vi "Test_read_memory.vi"() -> ()   [LabVIEW 2013]
uses:
  Input_5782/5782_Fast_PID_states.ctl
  <vilib>/Platform/TimedLoop/XDataNode/timing_clust.ctl
  <vilib>/Platform/TimedLoop/XDataNode/nitl_modes.ctl
  <vilib>/Platform/TimedLoop/XDataNode/wakeup.ctl
  <vilib>/rvi/FXPMathLib/FxpConvert/subVIs/nifxpmath_Convert_SimConfig.ctl
  <vilib>/fxp/LVFixedPointQuantizationPolicyTypeDef.ctl
  <vilib>/fxp/LVFixedPointOverflowPolicyTypeDef.ctl
  <vilib>/rvi/Emulation/niFpgaSctlEmulationGetInTimedLoop.vi
  <vilib>/rvi/Emulation/niFpgaEmulationReportErrorSimple.vi
  <vilib>/rvi/Emulation/niFpgaGetClockAttributes.vi
  <vilib>/rvi/eio/common/nirviEmuTemplateMethod_errors.vi
  <vilib>/rvi/Emulation/niFpgaCriticalErrorInLSC.vi
  <vilib>/rvi/FXPMathLib/FxpConvert/simVIs/DllFxpConvertTemp_sub.vi
  <vilib>/rvi/Memory/Memory_Emulation/nirvimemoryFastEmulationFpgaImpl.vi
  <instcachedir>/0/nirvimemoryFastEmulationFpgaImpl_5FBAB50466BC4C939F684F8805638BFC.lvgen/nirvimemoryFastEmulationFpgaImpl_5FBAB50466BC4C939F684F8805638BFC_003.vi
  <vilib>/rvi/DataTransferAndStorage/Container/Common/niFpgaContainerGetUniqueNameForEmu.vi
  <vilib>/rvi/Memory/Memory_Emulation/nirvimemoryFastEmulation.vi
  <vilib>/rvi/Memory/Memory_Emulation/nirvimemoryEmulation.vi
  <vilib>/rvi/interface/RandomDataEmulation/nirviRandomDataFPGAFIFO.vi
  <vilib>/rvi/interface/RandomDataEmulation/niFpgaRandomDataHandleErrors.vi
  <vilib>/Platform/TimedLoop/XDataNode/XDataNode.xnode
  <vilib>/eio/EIONode/EIONode.xnode
  <vilib>/rvi/FXPMathLib/FxpInterpret/XNode/nifxpmath_Interpret.xnode
  <vilib>/rvi/FXPMathLib/FxpConvert/XNode/nifxpmath_Convert.xnode
  <vilib>/rvi/DataTransferAndStorage/Container/XNode/niFpgaContainer.xnode
  <vilib>/rvi/interface/RandomDataEmulation/nirviRandomDataFpgaReadWriteTemplate.vi
  <vilib>/Platform/TimedLoop/XDataNode/XDNodeRunTimeDep.lvlib
panel:
  out "IO Module\\Trigger Input":bool
  in  "Trigger Acquisition":bool
  in  "IO Module\\AO Data Sync":bool=TRUE
  in  "IO Module\\SPI Write Data":u16
  out "IO Module\\SPI Read Data":u8
  in  "IO Module\\SPI Read":bool
  in  "IO Module\\SPI Write":bool
  in  "IO Module\\SPI Address":u16
  in  "IO Module\\SPI Device":u8
  out "IO Module\\SPI Idle":bool
  in  "User Command Commit":bool
  in  "User Command":u8
  out "User Command Idle":bool
  out "User Command Status":u8
  in  "User Data 0":u8
  in  "User Data 1":u8
  out "PLL Locked":bool
  out "User Error":bool
  out "Configured?":bool
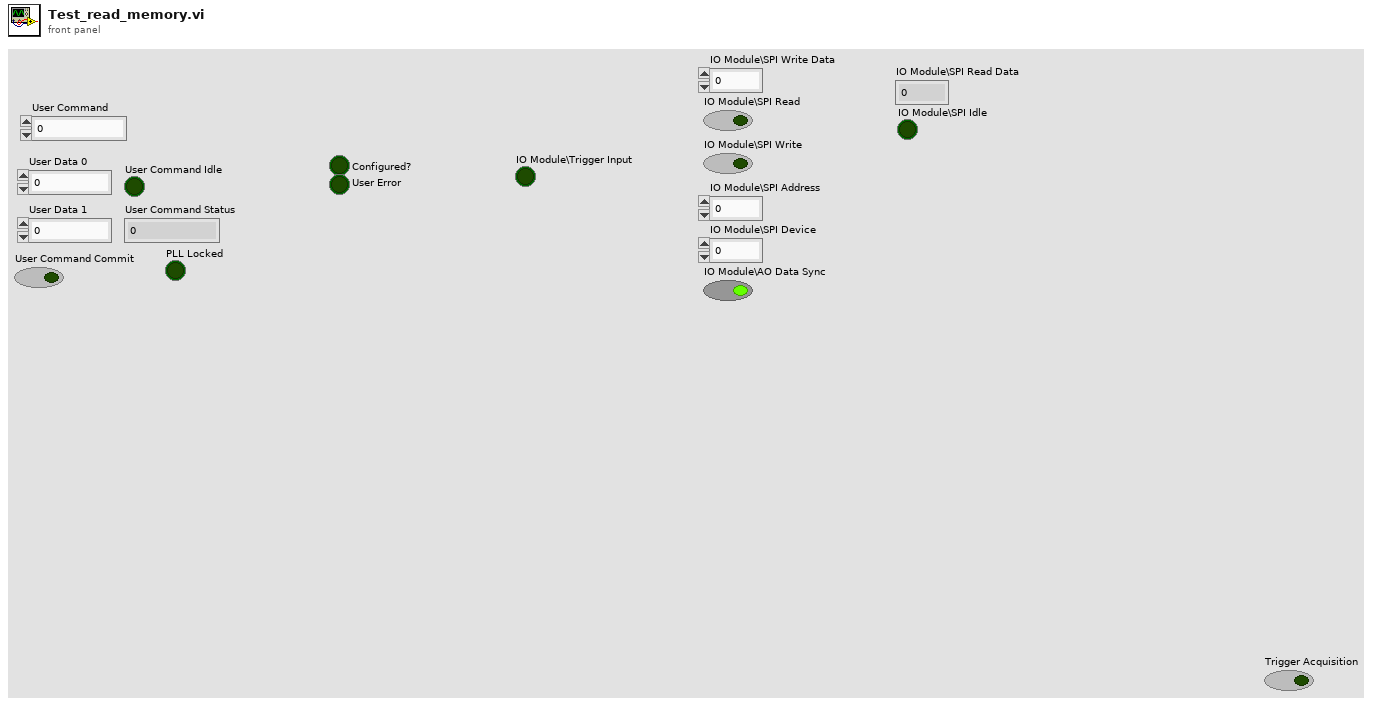
[diagram p1: front panel]
types:
  T1 = typedef "5782_Fast_PID_states.ctl" = enum8{"Wait for trigger", "Acquisition", "Send record length", "Wait for output", "Quiet period"}
  T2 = typedef "XDNodeRunTimeDep.lvlib/timing_clust.ctl" = cluster{"Expected End [f-1]":u64, "Actual End [f-1]":u64, "Finished Late? [f-1]":bool, "Expected End [i-1]":u64, "Actual End [i-1]":u64, "Finished Late? [i-1]":bool, "Expected Start [i]":u64, "Actual Start [i]":u64, "Expected Start [f]":u64, "Actual Start [f]":u64, "Source Name":string, "Structure Name":string, "Period":i64, "Deadline":i64, "Offset":i64, "Start":i64, "Priority":i32, "Timeout":i32, "Mode":T3, "Wakeup Reason":T4, "Error":errorcluster, "Source Type":string, "Secondary Source Type":string, "Global End Time":u64, "Global Start Time":u64, "Frame Duration":u64, "Iteration Duration":u64, "Assigned CPU":i32, "I/O Scan Engine Mode":u32}
  T3 = typedef "XDNodeRunTimeDep.lvlib/nitl_modes.ctl" = enum32{"No Change", "Process missed periods, maintain original phase", "Discard missed periods, maintain original phase", "Process missed periods, ignore original phase", "Discard missed periods, ignore original phase"}
  T4 = typedef "XDNodeRunTimeDep.lvlib/wakeup.ctl" = enum32{"Normal", "Aborted", "Asynchronous wakeup", "Timing source error", "Timed loop error", "Timeout"}
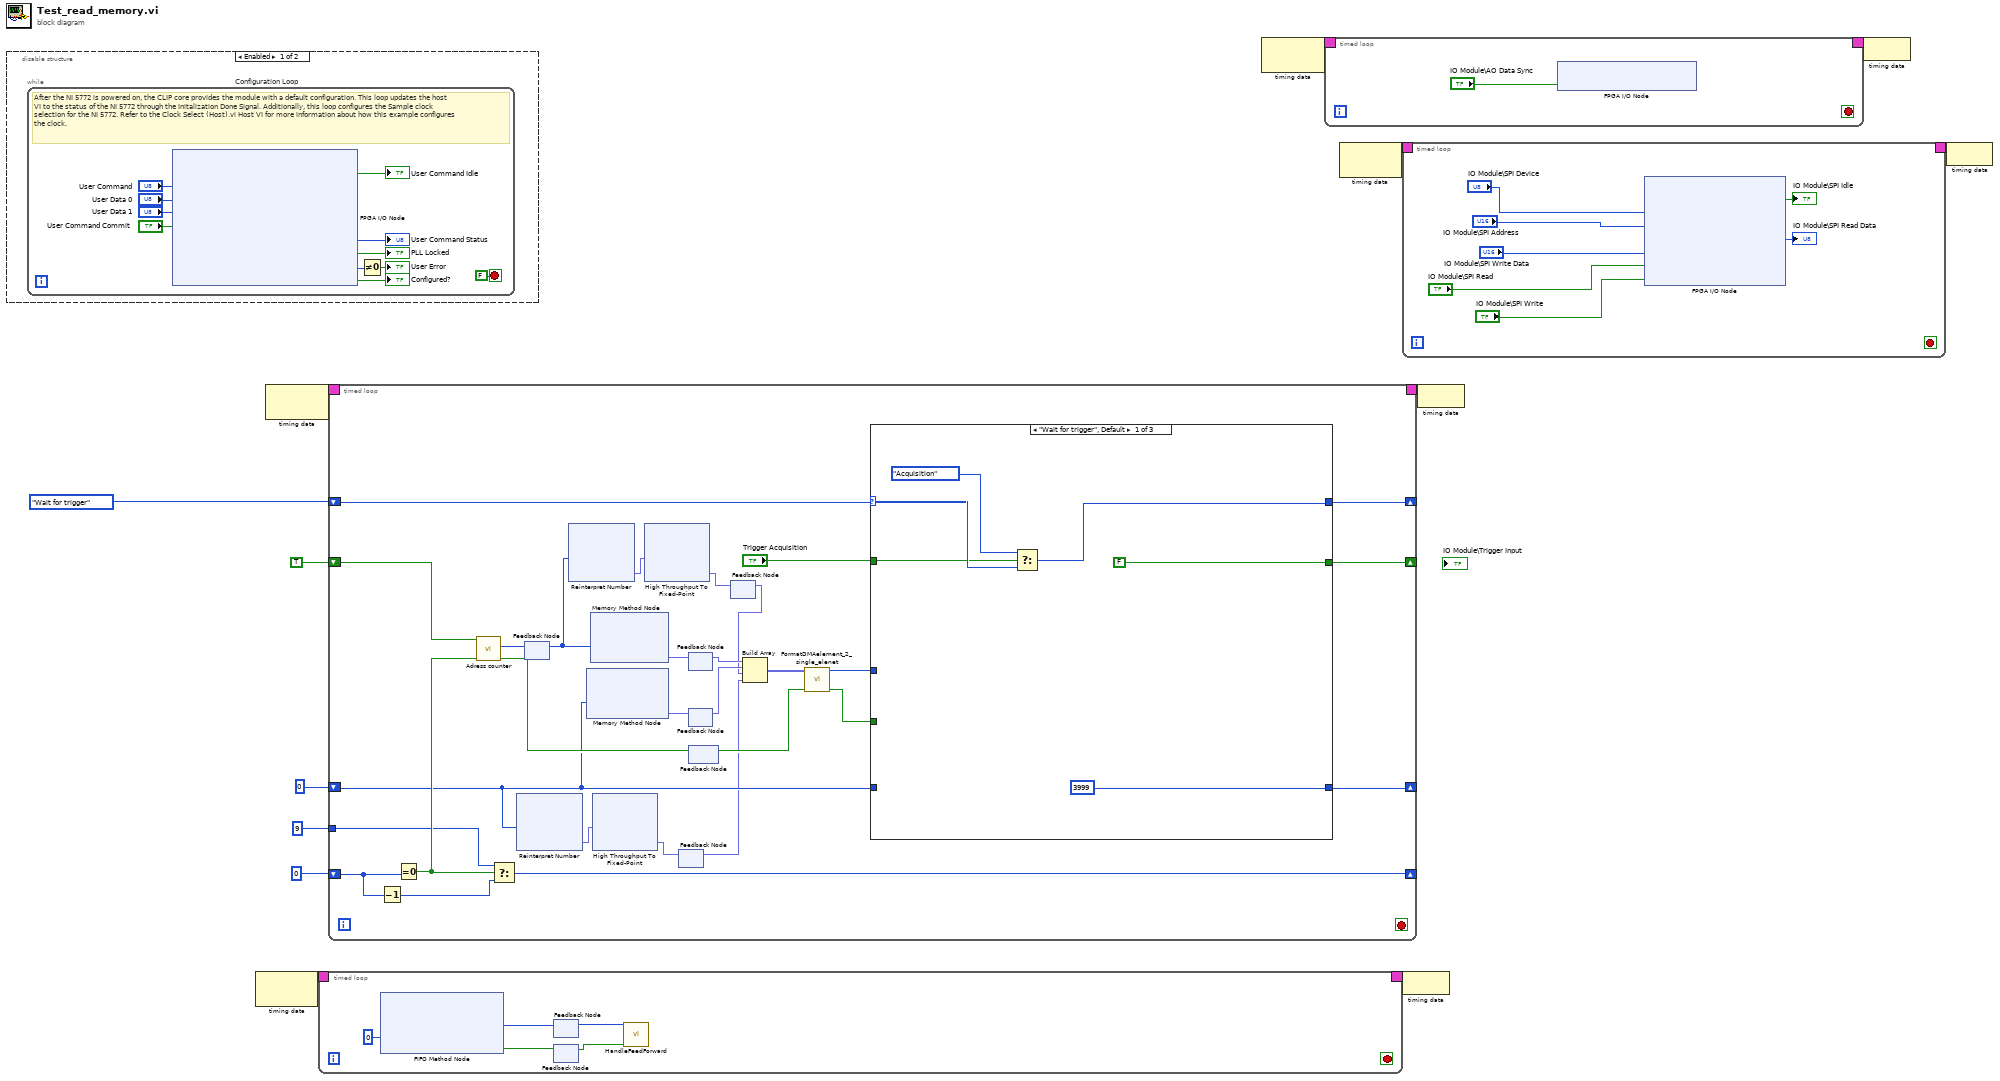
[diagram p0: block diagram]
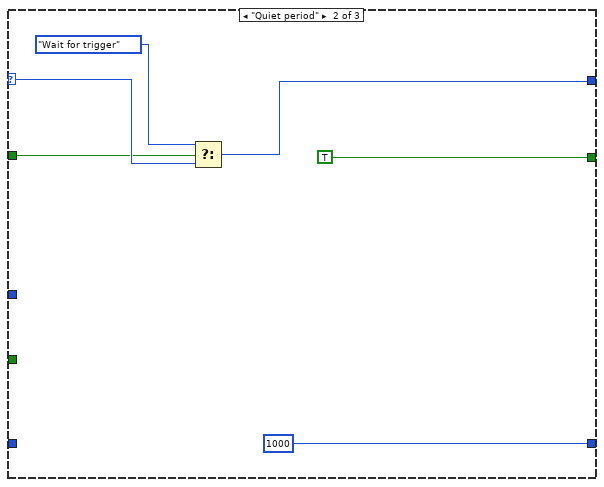
[diagram p2: hidden frame]
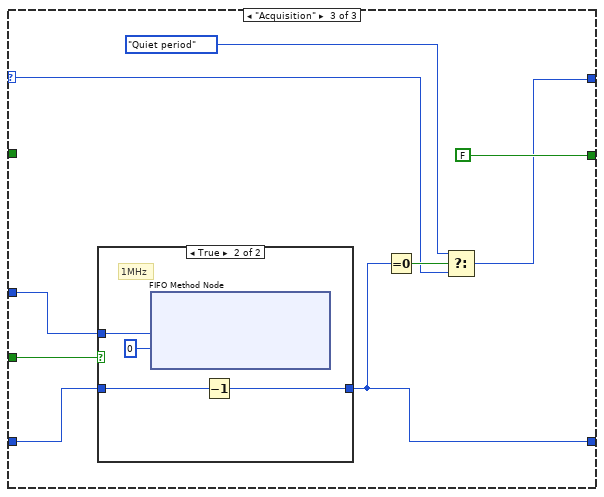
[diagram p3: hidden frame]
diagram:
  n1 = disable-structure shown="Enabled" {
    frame Enabled {
      n2 = while "Configuration Loop" {
        stop <- FALSE stop-if-true
        # "After the NI 5772 is powered on, the CLIP core provides the module with a default configuration. This loop updates the host VI to the status of the NI 5772 through the Initalization Done Signal. Additionally, this loop configures the Sample clock selection for the NI 5772. Refer to the Clock Select (Host).vi Host VI for more information about how this example configures the clock."
        n3 = xnode "FPGA I/O Node"("IO Module\\User Command"="User Command", "IO Module\\User Data 0"="User Data 0", "IO Module\\User Data 1"="User Data 1", "IO Module\\User Command Commit"="User Command Commit") -> ("IO Module\\User Command Idle"=→"User Command Idle":bool, "IO Module\\User Command Status"=→"User Command Status":u8, "IO Module\\PLL Locked"=→"PLL Locked":bool, "IO Module\\User Error"=w19:u8, "IO Module\\Initialization Done"=→"Configured?":bool)  [unwired: 9 in, 9 out]
        n4 = Not Equal To 0?(x=w19) -> (x != 0?=→"User Error":bool)
      }
    }
    frame Disabled {
    }
  }
  n5 = node-c288() -> (w13:T2)  [unwired: 1 in]
  n6 = node-c288() -> (w7:T2)  [unwired: 1 in]
  n7 = timed-loop {
    timing: w13 -> [_]
    timing-out: [_] -> w12
    stop <- _ stop-if-true
    n8 = xnode ("FIFO Method Node")("Timeout"=0) -> ("Element"=w28:u64, "Timed Out?"=w26:bool)  [unwired: 1 in, 1 out]
    n9 = feedback #1() -> (w27:u64)  [unwired: 1 in]
    n10 = feedback-in #1(w28) -> ()
    n11 = feedback #2() -> (w25:bool)  [unwired: 1 in]
    n12 = feedback-in #2(w26) -> ()
    n13 = call "HandleFeedForward.vi"("timed out"=w25, "Value"=w27) -> ()  [unwired: 10 in]
  }
  n14 = timed-loop {
    timing: w7 -> [_]
    timing-out: [_] -> w6
    shift-right: [w47] -> _
    shift-left: TRUE -> [w56]
    shift-right: [w51] -> _
    shift-left: u16 0 -> [w53]
    tunnel: u16 9 -> [w54]
    shift-right: [w48] -> _
    shift-left: 5782_Fast_PID_states."Wait for trigger" ("5782 states") -> [w50]
    shift-right: [w49] -> _
    shift-left: u32 0 -> [w33]
    stop <- _ stop-if-true
    n15 = Decrement(x=w53) -> (x-1=w52:u16)
    n16 = Equal To 0?(x=w53) -> (x = 0?=w55:bool)
    n17 = call "Adress counter.vi"("input valid"=w55, "Reset"=w56) -> ("output valid"=w60:bool, "Address"=w57:u32)  [unwired: 8 in]
    n18 = Select(t=w54, s=w55, f=w52) -> (s? t:f=w51:u16)
    n19 = xnode "Reinterpret Number"("x"=w33) -> ("y"=w34:fxp<+/-,32,32>)
    n20 = feedback #3() -> (w39:u32)  [unwired: 1 in]
    n21 = feedback-in #3(w57) -> ()
    n22 = xnode "Reinterpret Number"("x"=w39) -> ("y"=w38:fxp<+/-,32,32>)
    n23 = xnode ("Memory Method Node")("Address"=w33) -> ("Data"=w58:fxp<+/-,16,14>)  [unwired: 1 in, 1 out]
    n24 = xnode ("Memory Method Node")("Address"=w39) -> ("Data"=w59:fxp<+/-,16,14>)  [unwired: 1 in, 1 out]
    n25 = xnode ("High Throughput To Fixed-Point")("x"=w34) -> ("y"=w35:fxp<+/-,16,14>)
    n26 = xnode ("High Throughput To Fixed-Point")("x"=w38) -> ("y"=w37:fxp<+/-,16,14>)
    n27 = feedback #4() -> (w32:fxp<+/-,16,14>)  [unwired: 1 in]
    n28 = feedback-in #4(w35) -> ()
    n29 = feedback #5() -> (w45:fxp<+/-,16,14>)  [unwired: 1 in]
    n30 = feedback-in #5(w59) -> ()
    n31 = feedback #6() -> (w44:fxp<+/-,16,14>)  [unwired: 1 in]
    n32 = feedback-in #6(w58) -> ()
    n33 = feedback #7() -> (w43:bool)  [unwired: 1 in]
    n34 = feedback-in #7(w60) -> ()
    n35 = feedback #8() -> (w36:fxp<+/-,16,14>)  [unwired: 1 in]
    n36 = feedback-in #8(w37) -> ()
    n37 = Build Array(w45, w44, w36, w32) -> (w46:fxp<+/-,16,14>[])
    n38 = call "FormatDMAelement_2_single_elenet.vi"("valid in"=w43, "Data in"=w46) -> ("valid out"=w42:bool, "Element"=w41:u64)  [unwired: 8 in]
    n39 = case shown="\"Wait for trigger\", Default" w50 {
      selector: w50 -> [w108 w114 w119]
      tunnel: w33 -> [_ _ w125]
      tunnel: [u16 3999 u16 1000 w124] -> w49
      tunnel: [w107 w113 w117] -> w48
      tunnel: [FALSE TRUE FALSE] -> w47
      tunnel: w42 -> [_ _ w123]
      tunnel: w41 -> [_ _ w122]
      tunnel: "Trigger Acquisition" -> [w105 w111 _]
      frame "Wait for trigger", Default {
        n40 = Select(t=5782_Fast_PID_states."Acquisition" ("5782 states"), s=w105, f=w108) -> (s? t:f=w107:T1)
      }
      frame "Quiet period" {
        n41 = Select(t=5782_Fast_PID_states."Wait for trigger" ("5782 states"), s=w111, f=w114) -> (s? t:f=w113:T1)
      }
      frame "Acquisition" {
        n42 = case shown="True" w123 {
          tunnel: w122 -> [_ w130]
          tunnel: [w126 w127] -> w124
          tunnel: w125 -> [w126 w128]
          frame False {
          }
          frame True {
            # "1MHz"
            n43 = xnode ("FIFO Method Node")("Element"=w130, "Timeout"=0) -> ()  [unwired: 1 in, 2 out]
            n44 = Decrement(x=w128) -> (x-1=w127:u32)
          }
        }
        n45 = Equal To 0?(x=w124) -> (x = 0?=w120:bool)
        n46 = Select(t=5782_Fast_PID_states."Quiet period", s=w120, f=w119) -> (s? t:f=w117:T1)
      }
    }
  }
  n47 = node-c288() -> (w9:T2)  [unwired: 1 in]
  n48 = timed-loop {
    timing: w9 -> [_]
    timing-out: [_] -> w8
    stop <- _ stop-if-true
    n49 = xnode "FPGA I/O Node"("IO Module\\AO Data Sync"="IO Module\\AO Data Sync") -> ()  [unwired: 1 in, 1 out]
  }
  n50 = node-c288() -> (w11:T2)  [unwired: 1 in]
  n51 = timed-loop {
    timing: w11 -> [_]
    timing-out: [_] -> w10
    stop <- _ stop-if-true
    n52 = xnode "FPGA I/O Node"("IO Module\\SPI Device"="IO Module\\SPI Device", "IO Module\\SPI Address"="IO Module\\SPI Address", "IO Module\\SPI Write Data"="IO Module\\SPI Write Data", "IO Module\\SPI Read"="IO Module\\SPI Read", "IO Module\\SPI Write"="IO Module\\SPI Write") -> ("IO Module\\SPI Idle"=→"IO Module\\SPI Idle":bool, "IO Module\\SPI Read Data"=→"IO Module\\SPI Read Data":u8)  [unwired: 7 in, 7 out]
  }
  n53 = node-c288(w12) -> ()
  n54 = node-c288(w6) -> ()
  n55 = node-c288(w8) -> ()
  n56 = node-c288(w10) -> ()
